vi "ExtendedKalmanFilter_Predict.vi"(5 "f_Func":T1, 7 "F_Func_ExtraData":variant, 9 "dT_Seconds":dbl, 10 "U":T2, 11 "in UnscentedKalmanFiilter":T3) -> (0 "Error":bool, 3 "out UnscentedKalmanFiilter":T3)   [LabVIEW 2019, in "Trajectory_Library.lvlib"]
doc: "Creates a new LINEAR SYSTEM data cluster with the specified values. \n\n\nInputs: \n - XXX -- XXX.\n\nOutputs:\n - XXX -- XXX."
uses:
  Trajectory_Library.lvlib
  EXTENDED_KALMAN_FILTER.ctl
  <vilib>/Analysis/Matrix/Datatypes/RealMatrix.ctl
  BiFun_Matrix_FUNC_TYPE.ctl
  <vilib>/Analysis/7linalg.llb/Real Transpose Matrix.vi
  <vilib>/Analysis/baseanly.llb/Real A x B.vi
  Discretization_DiscretizeA.vi
  MatBuilder_Create.vi
  <vilib>/Analysis/Matrix/Numeric/Add/Add - RM,RM.vi
  <vilib>/Analysis/Matrix/Numeric/Multiply/Multiply.vi
  <vilib>/Analysis/Matrix/Numeric/Multiply/Multiply - RM,R.vi
  Matrix_Exp.vi
  <vilib>/Analysis/Matrix/NI_Matrix.lvlib
  <vilib>/Analysis/NI_AALBase.lvlib
  <vilib>/Analysis/NI_AALPro.lvlib
panel:
  # "State Estimate <Statess,1>"
  # "<States, States>"
  # "<States, States>"
  # "<Statess,  States>"
  # "<Outputs, Outputs>"
  # "State Estimate <Statess,1>"
  # "<States, States>"
  # "<States, States>"
  # "<Statess,  States>"
  # "<Outputs, Outputs>"
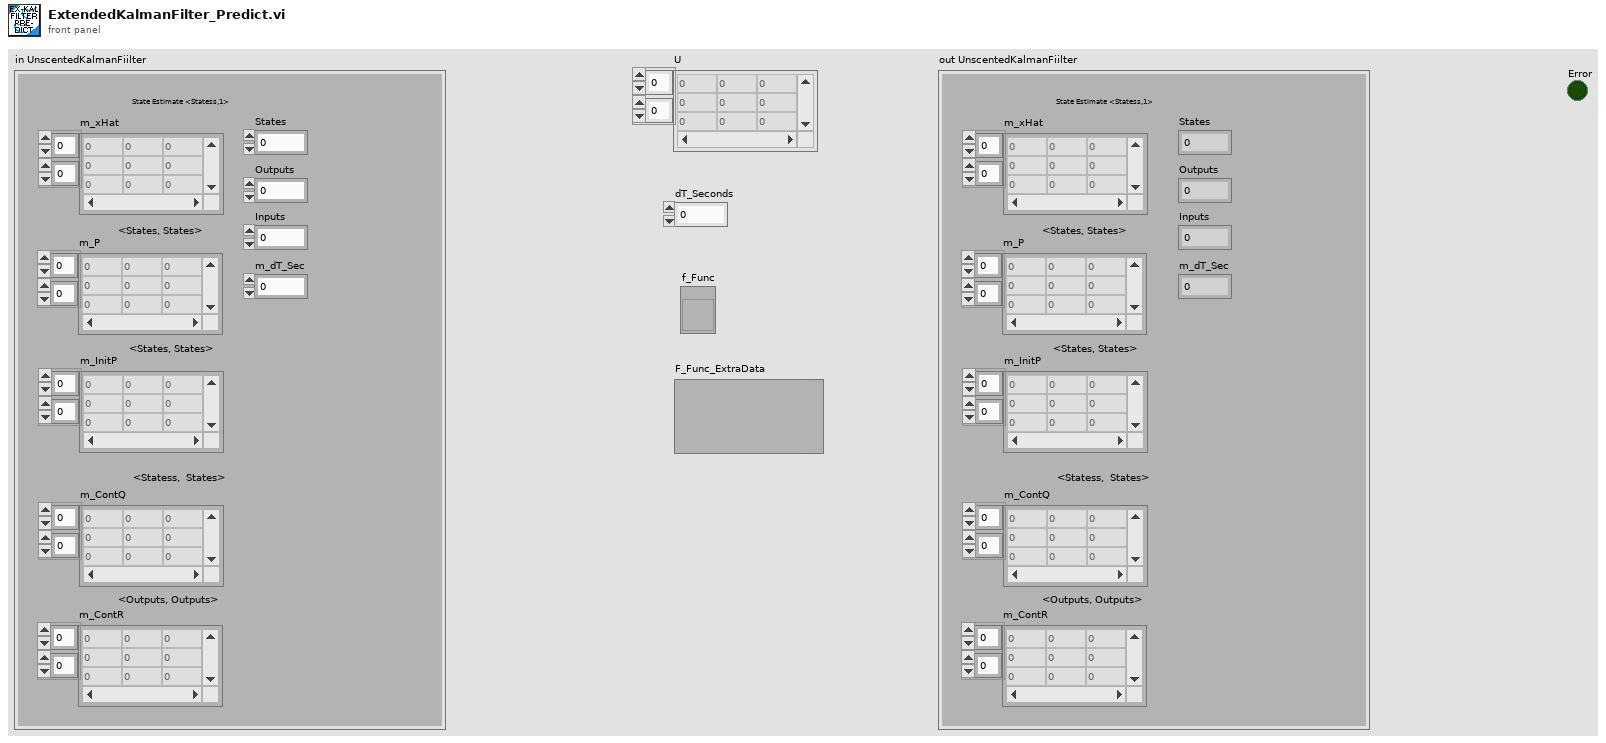
[diagram p1: front panel]
types:
  T1 = typedef "Trajectory_Library.lvlib/BiFun_Matrix_FUNC_TYPE.ctl" = refnum<vi>
  T2 = typedef "NI_Matrix.lvlib/RealMatrix.ctl" = dbl[][]
  T3 = typedef "Trajectory_Library.lvlib/EXTENDED_KALMAN_FILTER.ctl" = cluster{"m_P":T2, "m_xHat":T2, "States":i32, "Outputs":i32, "m_ContR":T2, "m_ContQ":T2, "m_dT_Sec":dbl, "Inputs":i32, "m_InitP":T2}
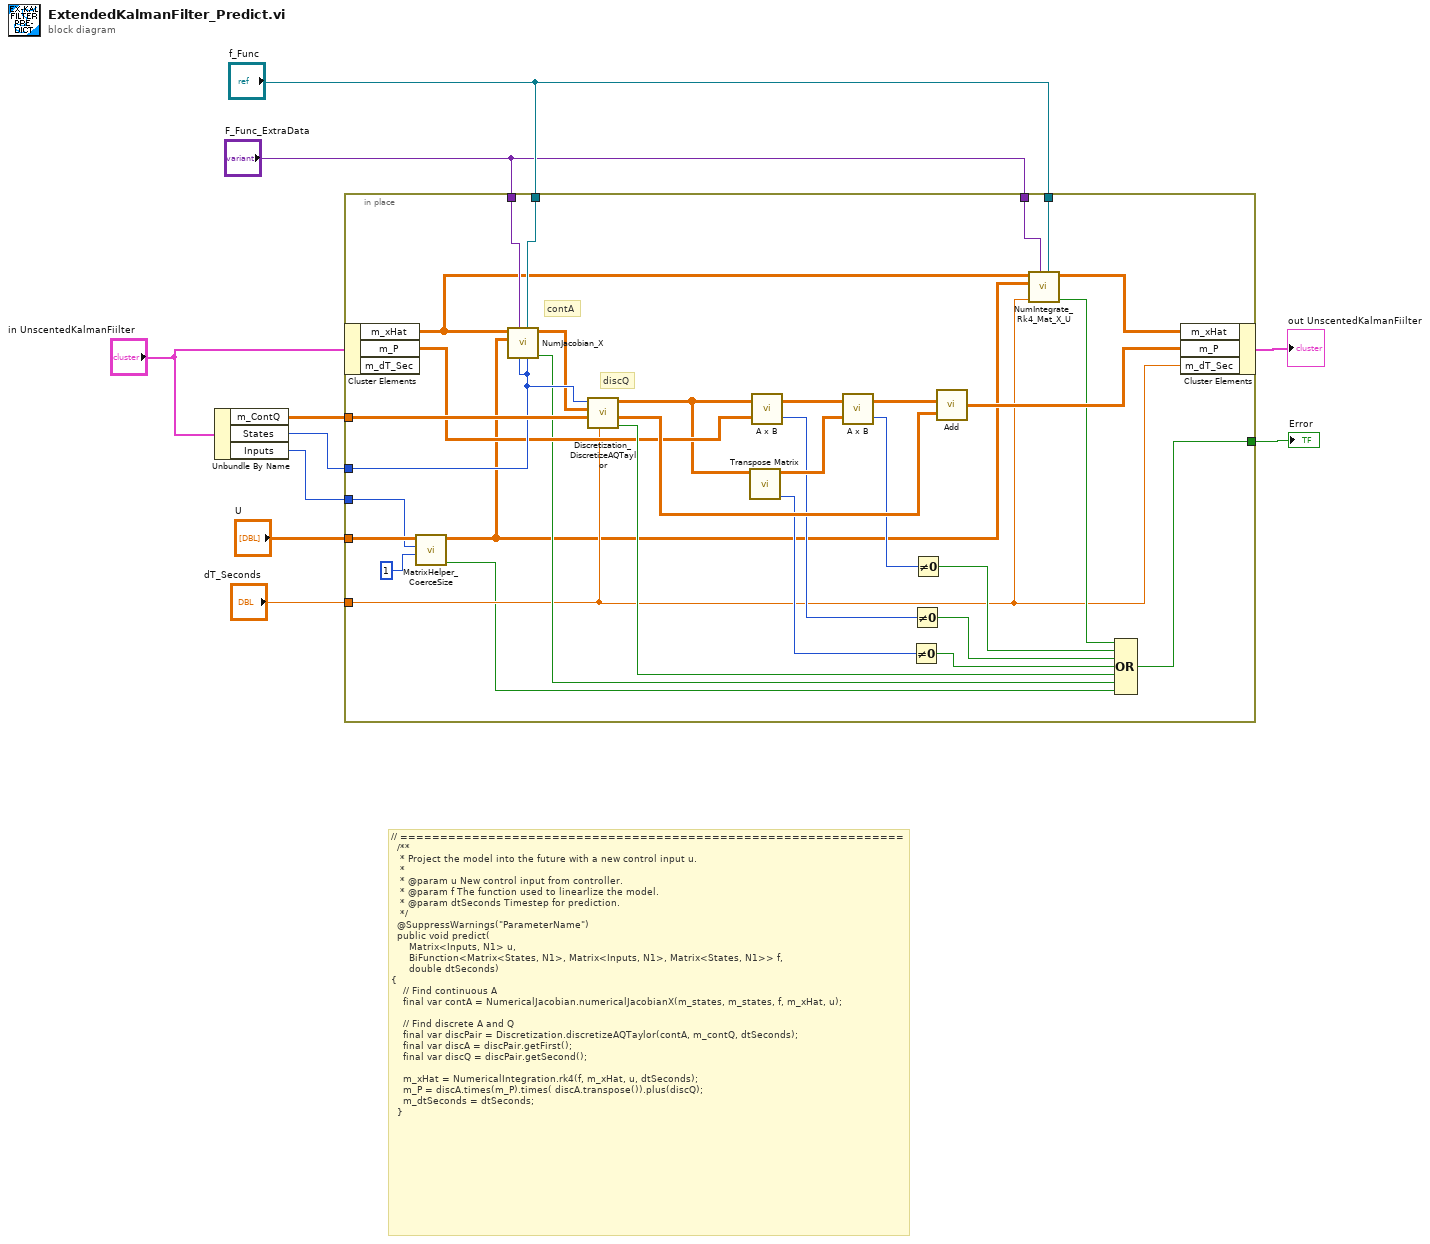
[diagram p0: block diagram]
diagram:
  # "// ===============================================================\n  /**\n   * Project the model into the future with a new control input u.\n   *\n   * @param u New control input from controller.\n   * @param f The function used to linearlize the model.\n   * @param dtSeconds Timestep for prediction.\n   */\n  @SuppressWarnings(\"ParameterName\")\n  public void predict(\n      Matrix<Inputs, N1> u,\n      BiFunction<Matrix<States, N1>, Matrix<Inputs, N1>, Matrix<States, N1>> f,\n      double dtSeconds) \n{\n    // Find continuous A\n    final var contA = NumericalJacobian.numericalJacobianX(m_states, m_states, f, m_xHat, u);\n\n    // Find discrete A and Q\n    final var discPair = Discretization.discretizeAQTaylor(contA, m_contQ, dtSeconds);\n    final var discA = discPair.getFirst();\n    final var discQ = discPair.getSecond();\n\n    m_xHat = NumericalIntegration.rk4(f, m_xHat, u, dtSeconds);\n    m_P = discA.times(m_P).times( discA.transpose()).plus(discQ);\n    m_dtSeconds = dtSeconds;\n  }"
  n1 = Unbundle By Name("in UnscentedKalmanFiilter") -> ("m_ContQ"=w8:T2, "States"=w6:i32, "Inputs"=w1:i32)
  n2 = in-place {
    in-place-border: "dT_Seconds" -> [w16]
    in-place-border: w8 -> [w42]
    in-place-border: "f_Func" -> [w41]
    in-place-border: "F_Func_ExtraData" -> [w40]
    in-place-border: "U" -> [w15]
    in-place-border: w6 -> [w37]
    in-place-border: "f_Func" -> [w39]
    in-place-border: "F_Func_ExtraData" -> [w38]
    in-place-border: [w23] -> w2
    in-place-border: w1 -> [w13]
    # "discQ"
    # "contA"
    n3 = in-place-cluster #1("in UnscentedKalmanFiilter") -> ("m_xHat"=w32:T2, "m_P"=w30:T2)  [unwired: 1 out]
    n4 = call "MatrixHelper_CoerceSize.vi"("Columns"=1, "Rows"=w13, "input matrix"=w15) -> ("Coerced"=w11:bool, "output matrix"=w14:T2)  [unwired: 7 in]
    n5 = call "NumJacobian_X.vi"("States"=w37, "F_FUNC"=w39, "Rows"=w37, "ExtraPassedData"=w38, "U"=w14, "X"=w32) -> ("Error"=w26:bool, "Result"=w36:T2)  [unwired: 4 in]
    n6 = call "Discretization_DiscretizeAQTaylor.vi"("dT_Seconds"=w16, "ContQ"=w42, "ContA"=w36, "States"=w37) -> ("Error"=w33:bool, "DiscQ"=w34:T2, "DiscA"=w29:T2)  [unwired: 5 in]
    n7 = call-poly <vilib>:"Transpose Matrix.vi"("Input Matrix"=w29) -> ("error"=w20:i32, "Matrix Transpose"=w27:T2)  [unwired: 9 in]
    n8 = call-poly <vilib>:"A x B.vi"("B"=w30, "A"=w29) -> ("error"=w22:i32, "A x B"=w28:T2)
    n9 = call-poly <vilib>:"A x B.vi"("B"=w27, "A"=w28) -> ("error"=w21:i32, "A x B"=w25:T2)
    n10 = Not Equal To 0?(x=w20) -> (x != 0?=w19:bool)
    n11 = Not Equal To 0?(x=w22) -> (x != 0?=w18:bool)
    n12 = Not Equal To 0?(x=w21) -> (x != 0?=w17:bool)
    n13 = call-poly <vilib>:"Add.vi"("Real Matrix B"=w34, "Real Matrix A"=w25) -> ("A + B"=w35:T2)
    n14 = call "NumIntegrate_Rk4_Mat_X_U.vi"("NumInt_RK4_Func_Type"=w41, "PassedData"=w40, "dT_Seconds"=w16, "U"=w14, "X"=w32) -> ("Error"=w24:bool, "OUTPUT"=w31:T2)  [unwired: 5 in]
    n15 = Compound Arithmetic op=OR(w24, w17, w18, w19, w33, w26, w11) -> (w23:bool)
    n16 = in-place-cluster #1("m_xHat"=w31, "m_P"=w35, "m_dT_Sec"=w16) -> (→"out UnscentedKalmanFiilter":T3)
  }
  "Error" <- w2
